vi "QUBE-Servo 2 Speed Control - myRIO.vi"() -> ()   [LabVIEW 2018]
uses:
  <vilib>/Simulation/Scripting/Companion Diagram/SimConfigNode/SimParams.ctl
  <vilib>/Simulation/Scripting/Companion Diagram/SimConfigNode/_simSolvers.ctl
  <vilib>/Simulation/Implementation/Shared/SIMSCR Execution Mode.ctl
  <vilib>/Platform/TimedLoop/XDataNode/timing_clust.ctl
  <vilib>/Platform/TimedLoop/XDataNode/nitl_modes.ctl
  <vilib>/Platform/TimedLoop/XDataNode/wakeup.ctl
  <vilib>/Simulation/Param Hierarchy/Typedefs/SIMPH Param Control Actions.ctl
  <vilib>/Quanser/Rapid Control Prototyping Toolkit/communications/basic/Basic Stream Send Mode.ctl
  <vilib>/Quanser/Rapid Control Prototyping Toolkit/communications/basic/Basic Stream Receive Mode.ctl
  <vilib>/Simulation/Implementation/Shared/NILVSim_ParamChanged.vi
  <vilib>/Simulation/Implementation/Shared/NILVSim_FinishedLate.vi
  <vilib>/Simulation/Implementation/Shared/NILVSIM_BeginStep.vi
  <vilib>/Simulation/Utility/Implementation/NILVSim Memory.llb/NILVSim Memory (core).vi
  <vilib>/Simulation/Utility/Implementation/SIM Halt.vi
  <vilib>/Simulation/ContinuousLinear/Implementation/NILVSim Transfer Function Direct.llb/SIM Transfer Function Direct (SISO).vi
  <vilib>/Simulation/SignalArithmetic/Implementation/NILVSim Gain.llb/SIM Gain (scalar).vi
  <vilib>/Simulation/Implementation/Shared/NILVSim_Manager.vi
  <vilib>/Utility/error.llb/Clear Errors.vi
  <vilib>/Simulation/Implementation/Shared/NILVSim_FinalizeModel.vi
  <vilib>/Simulation/Implementation/Shared/SIM Unbundle Sim Info.vi
  <vilib>/Simulation/Implementation/Shared/SIMSH Read Queue.vi
  <vilib>/Simulation/Implementation/Shared/NILVSim_Initialize.vi
  SubVIs/Hardware/QUBE2 RW.vi
  <vilib>/Simulation/Utility/Implementation/NILVSim Get Time and IsAcceptedStep.vi
  <vilib>/Simulation/Implementation/Shared/NILVSim_GetModelError.vi
  <vilib>/Simulation/Implementation/Shared/SIM Bundle Sim Info.vi
  <vilib>/Simulation/Scripting/Companion Diagram/SimConfigNode/SimDog.xnode
  SubVIs/Speed_PI_Control_Sim.vi
  <vilib>/Quanser/Rapid Control Prototyping Toolkit/communications/basic/_TypeSpecific/CL Comm Basic Stream Server (1D DBL).vi
  <vilib>/Quanser/Rapid Control Prototyping Toolkit/communications/basic/CL Comm Basic Stream Server.vi
  <vilib>/Platform/TimedLoop/XDataNode/XDataNode.xnode
  <vilib>/Simulation/Implementation/XNodeFramework/SimXNode/SimX.xnode
  <vilib>/Platform/TimedLoop/XDataNode/XDNodeRunTimeDep.lvlib
  <vilib>/Simulation/Implementation/Shared/NI_SIM_Implementation.lvlib
panel:
  out "Error":errorcluster
  in  "Halt?":bool
  out "Connection":T1(ring)
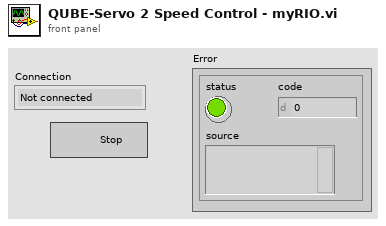
[diagram p1: front panel]
types:
  T1 = enum8{"Not connected", "Connecting...", "Connected", "Closing..."}
  T2 = typedef "QFLEX myRIO.ctl" = cluster{"Error":errorcluster, "CS DO Ref":T3, "SPI Ref":T10}
  T3 = typedef "DIO.lvlib/DIO Reference.ctl" = cluster{"myRIO Reference":T4, "DIO Channels List":T8}
  T4 = typedef "myRIO Generic Hardware Reference.ctl" = cluster{"myRIO Model":T5, "myRIO Hardware Reference":T6}
  T5 = typedef "Hardware Version Enum.ctl" = enum16{"Unknown", "myRIO-1900", "myRIO-1950", "roboRIO", "NI ELVIS RIO CM", "ELVIS III"}
  T6 = typedef "myRIO v1.0 Reference.ctl" = cluster{"Generic FPGA Reference":T7, "Allow multiple opens":bool}
  T7 = typedef "Generic FPGA Reference.ctl" = refnum<k20>
  T8 = typedef "DIO Channels List.ctl" = T9[]
  T9 = typedef "DIO Channels Enum.ctl" = enum16{"Not Connected", "C/DIO0", "C/DIO1", "C/DIO2", "C/DIO3", "C/DIO4", "C/DIO5", "C/DIO6", "C/DIO7", "A/DIO0", "A/DIO1", "A/DIO2", "A/DIO3", "A/DIO4", "A/DIO5", "A/DIO6", "A/DIO7", "A/DIO8", "A/DIO9", "A/DIO10", "A/DIO11", "A/DIO12", "A/DIO13", "A/DIO14", "A/DIO15", "A/DIO16", "A/DIO17", "A/DIO18", "A/DIO19", "B/DIO0", "B/DIO1", "B/DIO2", "B/DIO3", "B/DIO4", "B/DIO5", "B/DIO6", "B/DIO7", "B/DIO8", "B/DIO9", "B/DIO10", "B/DIO11", "B/DIO12", "B/DIO13", "B/DIO14", "B/DIO15", "B/DIO16", "B/DIO17", "B/DIO18", "B/DIO19", "LED0", "LED1", "LED2", "LED3", "Button0", "DIO/DIO0", "DIO/DIO1", "DIO/DIO2", "DIO/DIO3", "DIO/DIO4", "DIO/DIO5", "DIO/DIO6", "DIO/DIO7", "DIO/DIO8", "DIO/DIO9", "SPI/CS0", "SPI/CS1", "SPI/CS2", "SPI/CS3", "LED RADIO (Green)", "LED RADIO (Red)", "LED COMM (Green)", "LED COMM (Red)", "LED MODE (Green)", "LED MODE (Red)"}
  T10 = typedef "SPI.lvlib/SPI Reference.ctl" = cluster{"myRIO Reference":T4, "SPI Channels Enum":T11, "SPI Configuration":T12}
  T11 = typedef "SPI Channels Enum.ctl" = enum16{"Not Connected", "A/SPI", "B/SPI", "SPI/SPI"}
  T12 = typedef "SPI.lvlib/SPI Configuration.ctl" = cluster{"Frequency [Hz]":dbl, "Clock Phase":T13, "Clock Polarity":T14, "Data Direction":T15, "Frame Length":T16}
  T13 = typedef "SPI Clock Phase.ctl" = enum8{"Leading", "Trailing"}
  T14 = typedef "SPI Clock Polarity.ctl" = enum8{"Low", "High"}
  T15 = typedef "SPI Data Direction.ctl" = enum8{"Most significant bit first", "Least significant bit first"}
  T16 = typedef "SPI Frame Length.ctl" = u8
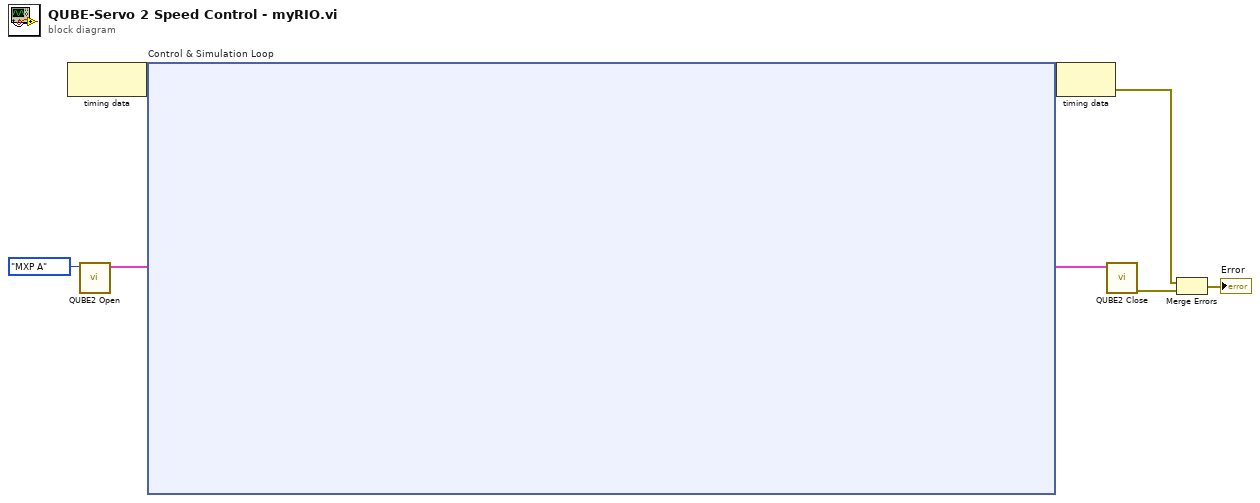
[diagram p0: block diagram]
diagram:
  n1 = node-c288() -> (w8:variant)  [unwired: 1 in]
  n2 = call "QUBE2 Open.vi"("Connector"=enum16{"MXP A", "MXP B"}."MXP A") -> ("QFLEX Cluster Out"=w5:T2)  [unwired: 10 in]
  n3 = node-c254 "Control & Simulation Loop"(w8, w5) -> (w7:variant, w4:T2)
  n4 = node-c288(w7) -> (w3:errorcluster)
  n5 = call "QUBE2 Close.vi"("QFLEX Cluster In"=w4) -> ("error out"=w2:errorcluster)  [unwired: 10 in]
  n6 = Merge Errors(w3, w2) -> (→"Error":errorcluster)
